vi "PID elapsed time.vi"(13 "reset":bool) -> (8 "elapsed time (ms)":u32, 15 "elaspsed time (sec)":dbl)   [LabVIEW 2019]
panel:
  # "this is a one shot with an USR, and a first call flag\n\nevery time you run it by hitting the run button above,\nit is the first call, thus it outputs zero\n\nit only works properly if called from above, so open\nthis fp first, and watch it while the main program is running it"
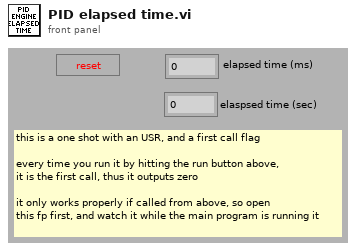
[diagram p1: front panel]
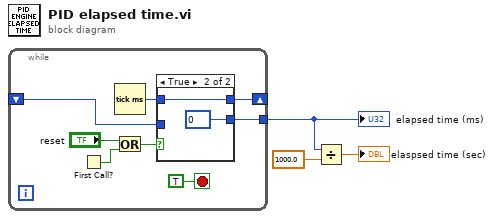
[diagram p0: block diagram]
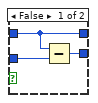
[diagram p2: hidden frame]
diagram:
  n1 = while {
    shift-left: _ -> [w8]
    shift-right: [w9] -> _
    tunnel: [w11] -> w3
    stop <- TRUE stop-if-true
    n2 = First Call?() -> (First Call?: T/F=w5:bool)
    n3 = Tick Count (ms)() -> (millisecond timer value=w7:u32)
    n4 = Or(x="reset", y=w5) -> (x .or. y?=w4:bool)
    n5 = case shown="True" w4 {
      tunnel: [w14 u32 0 ("current time (sec)")] -> w11
      tunnel: [w12 w15] -> w9
      tunnel: w8 -> [w13 _]
      tunnel: w7 -> [w12 w15]
      frame False {
        n6 = Subtract(x=w12, y=w13) -> (x-y=w14:u32)
      }
      frame True {
      }
    }
  }
  "elapsed time (ms)" <- w3
  n7 = Divide(x=w3, y=1000.0) -> (x/y=→"elaspsed time (sec)":dbl)
